vi "Application_regulation_numerique_AhmedAmrani.vi"() -> ()   [LabVIEW 2012]
uses:
  <vilib>/addons/Control Design/_Model Construction/Model Creation.llb/Model Creation SubVI/cd_Create Transfer Function Model.vi
  <vilib>/addons/Control Design/_Utility/Model Viewer.llb/Model Viewer SubVI/cd_Draw Transfer Function Equation (TF).vi
  <vilib>/addons/Control Design/_Utility/NI_CD_Model Viewer.lvlib
  <vilib>/addons/Control Design/_Model Construction/NI_LinSys_Model Creation.lvlib
panel:
  out "Systeme 2":picture
  out "Systeme":picture
  in  "chemin système flou":path=path "E:/cours td 3/automatique avancee/devoir/controlleur_flou_AhmedAmrani.fs"
  in  "Kr":dbl=1.0
  out "Erreur":dbl
  out "Feedback":enum32{" 1", " 2"}(tab)
  out "Controlleur":enum32{"1", "2", "3"}(tab)
  in  "Kp":dbl=9.855
  in  "Ti":dbl=2.8224
  in  "Td":dbl=0.6982
  in  "Valider paramètres":bool
  out "Type de controlleur":string
  out "Type de boucle":string
  out "Sortie":dbl
  in  "Valider perturbation":bool
  in  "Perturbation":dbl
  in  "a2p":dbl=1.0
  in  "a1p":dbl=1.0
  in  "a0p":dbl=1.0
  in  "b0p":dbl=1.0
  in  "Periode d'échant.":dbl=0.01
  in  "a2":dbl=1.0
  in  "a1":dbl=1.0
  in  "a0":dbl=1.0
  in  "b0":dbl=1.0
  in  "Controlleur numérique":bool=TRUE
  out "Commande":dbl
  in  "Remise  à zéro":bool
  in  "Stop":bool
  in  "Boucle \nfermée":bool=TRUE
  in  "Valider consigne":bool
  in  "consigne":dbl
  out "Waveform Chart":cluster{"u_n":dbl, dbl, "y_n":dbl}(graph)
  # "Ahmed Amrani Akdi - 3ème année GEMI FSTT - Dept génie électrique - automatique avancée\nDevoir : Simulation de la boucle de régulation d’un système de deuxième ordre avec perturbation avec choix du régulateur (PID ou flou) sous Labview"
  # "FT Perturbation"
  # "Système"
  # "Boucle ouverte"
  # "Controlleur Flou"
  # "Gain de retour"
  # "Mettez le chemin du fichier  .fs du controlleur flou."
  # "PID"
  # "En choisissant Ti = 0, le controlleur devient PD"
  # "Controlleur flou"
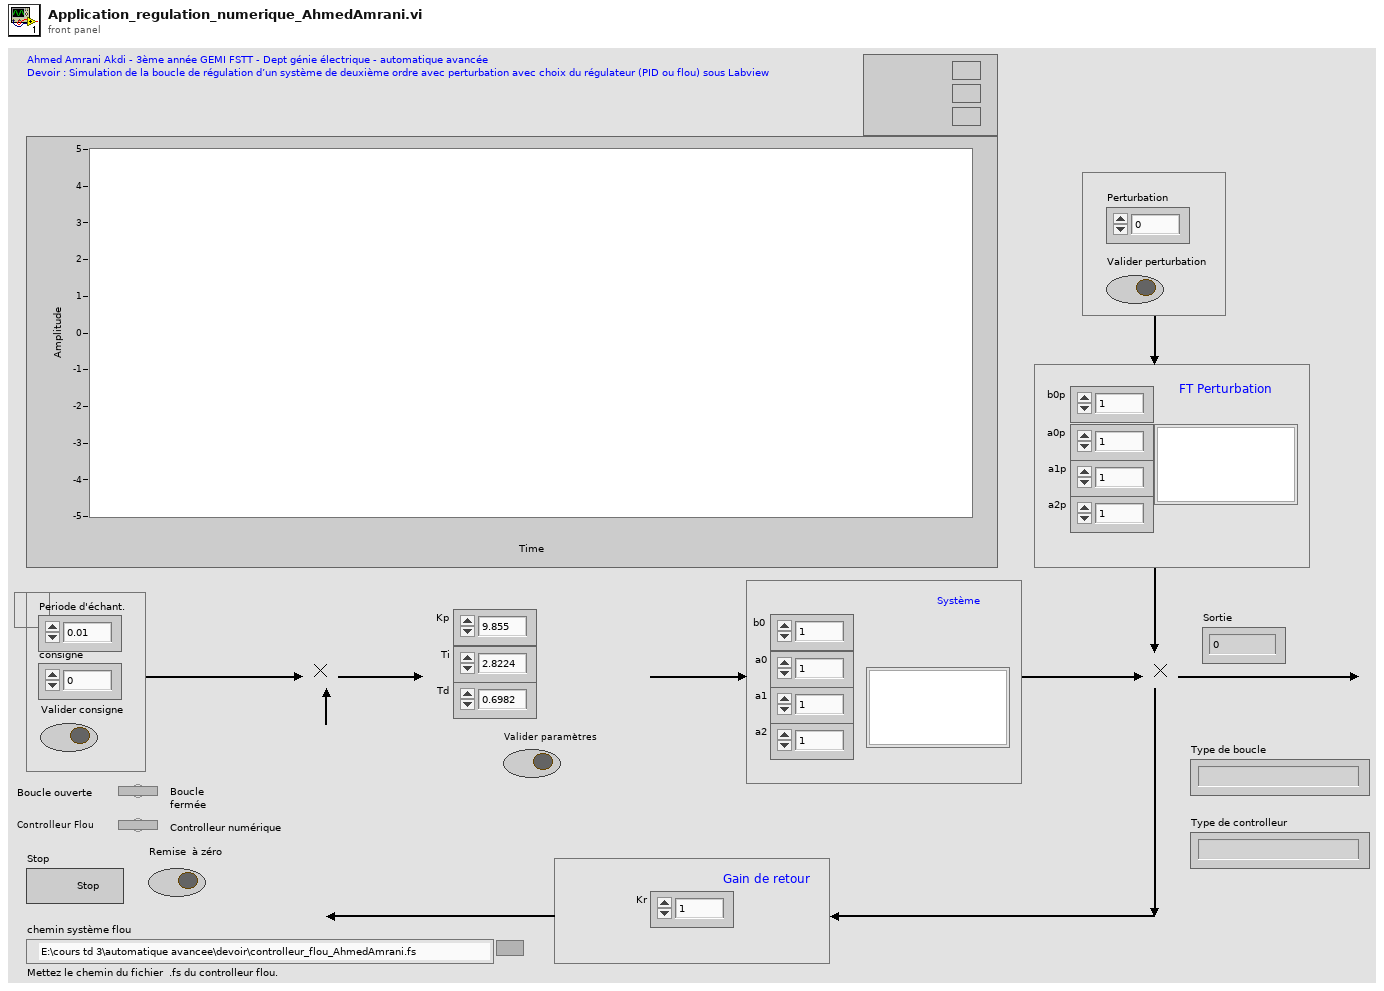
[diagram p1: front panel]
types:
  T1 = typedef "NI_LinSys_Model Typedefs.lvlib/CD Transfer Function Model (MIMO).ctl" = cluster{"properties":T2, "transfer function(s)":T3[][]}
  T2 = typedef "NI_LinSys_Model Typedefs.lvlib/CD General Elements.ctl" = cluster{"Model name":string, "Input names":string[], "Output names":string[], "Input Delays":dbl[], "Output Delays":dbl[], "Sampling Time":dbl, "Notes":string}
  T3 = typedef "NI_LinSys_Model Typedefs.lvlib/CD Transfer Function Model (SISO).ctl" = cluster{"Numerator":dbl[], "Denominator":dbl[], "delay":dbl}
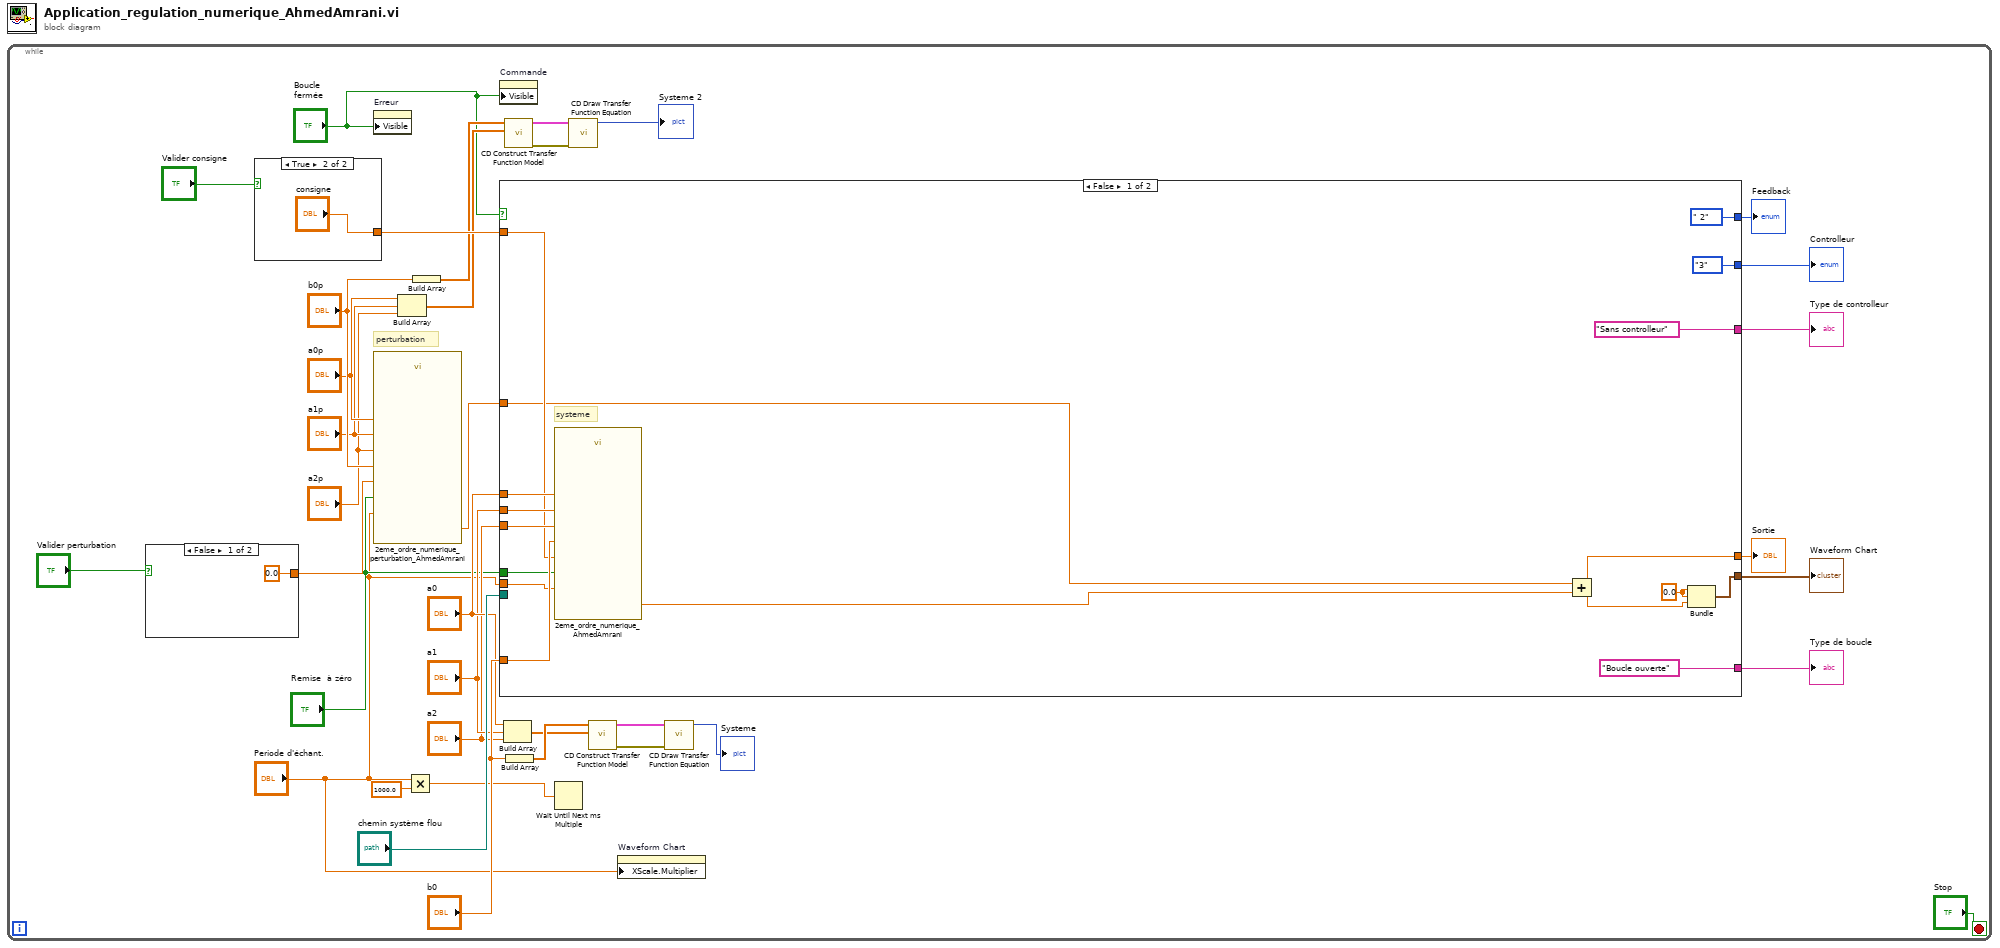
[diagram p0: block diagram]
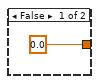
[diagram p2: hidden frame]
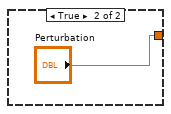
[diagram p3: hidden frame]
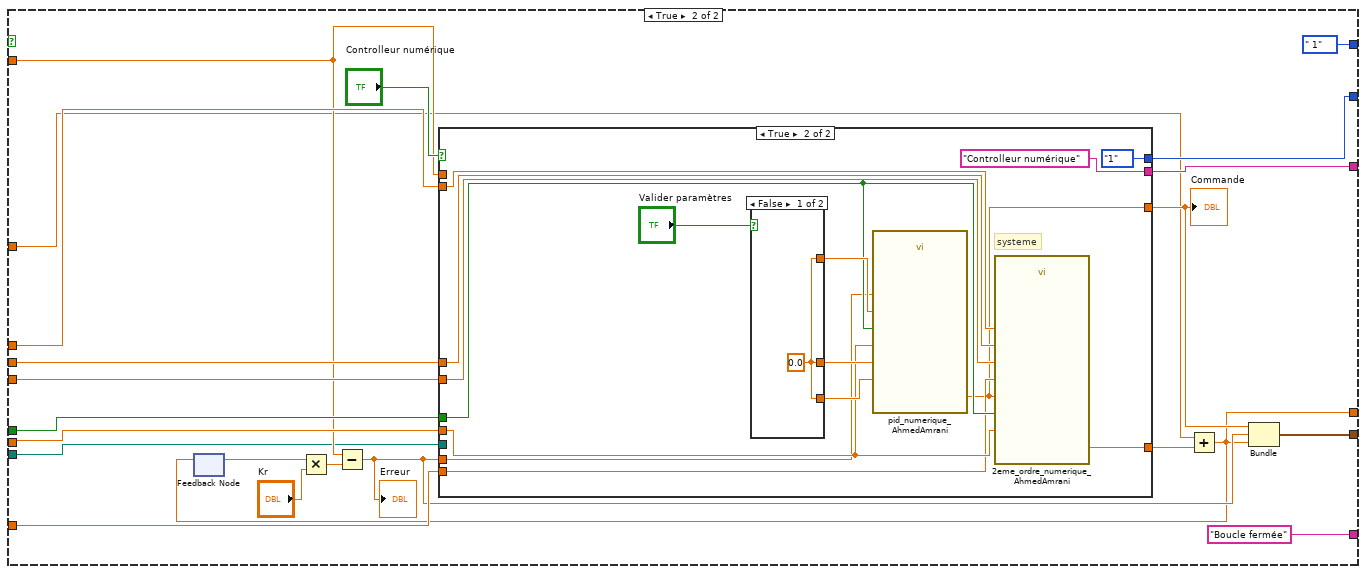
[diagram p4: hidden frame]
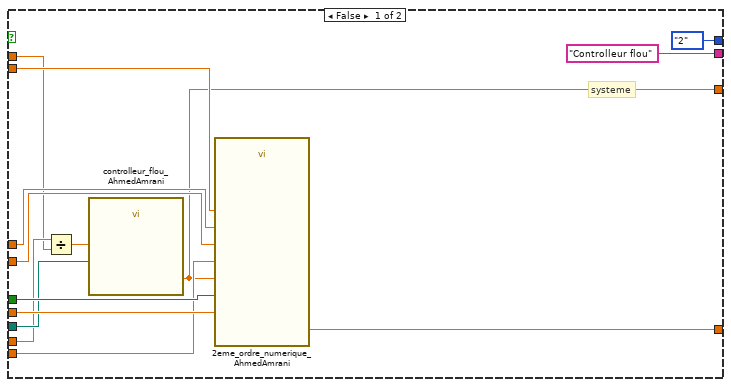
[diagram p5: hidden frame]
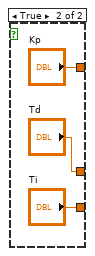
[diagram p6: hidden frame]
diagram:
  n1 = while {
    stop <- "Stop" stop-if-true
    # "perturbation"
    n2 = case shown="False" "Valider perturbation" {
      tunnel: [0.0 ("Perturbation") "Perturbation"] -> w16
      frame False {
      }
      frame True {
      }
    }
    n3 = case shown="True" "Valider consigne" {
      tunnel: [0.0 ("consigne") "consigne"] -> w34
      frame False {
      }
      frame True {
      }
    }
    n4 = property on="Erreur" class="DigNum (strict)"("Visible"="Boucle \nfermée") -> ()  [unwired: 2 in, 2 out]
    n5 = call "2eme_ordre_numerique_perturbation_AhmedAmrani.vi"("RAZ"="Remise  à zéro", "e_n"=w16, "T"="Periode d'échant.", "a2"="a2p", "a1"="a1p", "a0"="a0p", "b0"="b0p") -> ("y_n"=w15:dbl)  [unwired: 4 in]
    n6 = Build Array("a0p", "a1p", "a2p") -> (w11:dbl[])
    n7 = Multiply(x="Periode d'échant.", y=1000.0) -> (x*y=w2:dbl)
    n8 = Build Array("b0p") -> (w10:dbl[])
    n9 = property on="Commande" class="DigNum (strict)"("Visible"="Boucle \nfermée") -> ()  [unwired: 2 in, 2 out]
    n10 = case shown="False" "Boucle \nfermée" {
      tunnel: "Remise  à zéro" -> [w46 w68]
      tunnel: "a2" -> [w52 w78]
      tunnel: "a1" -> [w51 w77]
      tunnel: "a0" -> [w50 w76]
      tunnel: "b0" -> [w49 w75]
      tunnel: w34 -> [w48 w65]
      tunnel: "Periode d'échant." -> [w47 w74]
      tunnel: [enum32{" 1", " 2"}." 2" ("Tab Control 2") enum32{" 1", " 2"}." 1" ("Tab Control 2")] -> w33
      tunnel: ["Boucle ouverte" ("Type de boucle") "Boucle fermée" ("Type de boucle")] -> w32
      tunnel: ["Sans controlleur" ("Type de controlleur") w69] -> w31
      tunnel: [enum32{"1", "2", "3"}."3" ("Tab Control") w71] -> w30
      tunnel: [w42 w57] -> w29
      tunnel: [w45 w62] -> w28
      tunnel: "chemin système flou" -> [_ w60]
      tunnel: w15 -> [w43 w58]
      frame False {
        w44 = 0.0
        # "systeme"
        n11 = call "2eme_ordre_numerique_AhmedAmrani.vi"("RAZ"=w46, "e_n"=w48, "T"=w47, "a2"=w52, "a1"=w51, "a0"=w50, "b0"=w49) -> ("y_n"=w41:dbl)  [unwired: 4 in]
        n12 = Add(x=w43, y=w41) -> (x+y=w42:dbl)
        n13 = Bundle(w44, w44, w42) -> (w45:cluster{dbl, dbl, dbl})  [unwired: 1 in]
      }
      frame True {
        n14 = feedback #1() -> (w61:dbl)  [unwired: 1 in]
        n15 = Multiply(x=w61, y="Kr") -> (x*y=w66:dbl)
        n16 = Subtract(x=w65, y=w66) -> (x-y=w63:dbl)
        "Erreur" <- w63
        n17 = case shown="True" "Controlleur numérique" {
          tunnel: w74 -> [w89 w103]
          tunnel: w68 -> [w88 w104]
          tunnel: w78 -> [w87 w102]
          tunnel: w77 -> [w86 w101]
          tunnel: w76 -> [w85 w100]
          tunnel: w75 -> [w84 w99]
          tunnel: w65 -> [w80 _]
          tunnel: [enum32{"1", "2", "3"}."2" ("Tab Control") enum32{"1", "2", "3"}."1" ("Tab Control")] -> w71
          tunnel: ["Controlleur flou" ("Type de controlleur") "Controlleur numérique" ("Type de controlleur")] -> w69
          tunnel: [w90 w96] -> w59
          tunnel: w63 -> [w81 w94]
          tunnel: [w82 w95] -> w64
          tunnel: w60 -> [w83 _]
          frame False {
            # "systeme"
            n18 = Divide(x=w81, y=w80) -> (x/y=w79:dbl)
            n19 = call "controlleur_flou_AhmedAmrani.vi"("file path"=w83, "e_n"=w79) -> ("u_n"=w82:dbl)  [unwired: 9 in]
            n20 = call "2eme_ordre_numerique_AhmedAmrani.vi"("RAZ"=w88, "e_n"=w82, "T"=w89, "a2"=w87, "a1"=w86, "a0"=w85, "b0"=w84) -> ("y_n"=w90:dbl)  [unwired: 4 in]
          }
          frame True {
            # "systeme"
            n21 = case shown="False" "Valider paramètres" {
              tunnel: [w108 "Td"] -> w107
              tunnel: [w108 "Ti"] -> w106
              tunnel: [w108 "Kp"] -> w105
              frame False {
                w108 = 0.0 ("Kp")
              }
              frame True {
              }
            }
            n22 = call "pid_numerique_AhmedAmrani.vi"("RAZ"=w104, "e_n"=w94, "T"=w103, "Td"=w107, "Ti"=w106, "Kp"=w105) -> ("u_n"=w95:dbl)  [unwired: 5 in]
            n23 = call "2eme_ordre_numerique_AhmedAmrani.vi"("RAZ"=w104, "e_n"=w95, "T"=w103, "a2"=w102, "a1"=w101, "a0"=w100, "b0"=w99) -> ("y_n"=w96:dbl)  [unwired: 4 in]
          }
        }
        "Commande" <- w64
        n24 = Add(x=w58, y=w59) -> (x+y=w57:dbl)
        n25 = feedback-in #1(w57) -> ()
        n26 = Bundle("u_n"=w64, w63, w57) -> (w62:cluster{"u_n":dbl, dbl, dbl})  [unwired: 1 in]
      }
    }
    "Type de boucle" <- w32
    "Type de controlleur" <- w31
    "Feedback" <- w33
    "Controlleur" <- w30
    "Sortie" <- w29
    "Waveform Chart" <- w28
    n27 = Build Array("a0", "a1", "a2") -> (w19:dbl[])
    n28 = call-poly <vilib>:"CD Construct Transfer Function Model.vi"("Denominator"=w11, "Numerator"=w10) -> ("error out"=w14:errorcluster, "Transfer Function Model"=w13:T1)  [unwired: 8 in]
    n29 = Build Array("b0") -> (w23:dbl[])
    n30 = Wait Until Next ms Multiple(millisecond multiple=w2) -> ()  [unwired: 1 out]
    n31 = call-poly <vilib>:"CD Draw Transfer Function Equation.vi"("error in (no error)"=w14, "Transfer Function Model"=w13) -> ("Equation"=→"Systeme 2":picture)  [unwired: 7 in, 2 out]
    n32 = call-poly <vilib>:"CD Construct Transfer Function Model.vi"("Denominator"=w19, "Numerator"=w23) -> ("error out"=w26:errorcluster, "Transfer Function Model"=w25:T1)  [unwired: 8 in]
    n33 = property on="Waveform Chart" class="WFChart (strict)"("XScale.Multiplier"="Periode d'échant.") -> ()  [unwired: 2 in, 2 out]
    n34 = call-poly <vilib>:"CD Draw Transfer Function Equation.vi"("error in (no error)"=w26, "Transfer Function Model"=w25) -> ("Equation"=→"Systeme":picture)  [unwired: 7 in, 2 out]
  }
